vi "TestFindFaces.vi"() -> ()   [LabVIEW 2017]
uses:
  <vilib>/Enthought/Python Integration Toolkit/api/Console Visibility.ctl
  FindFaces_IMAQ.vi
  FindEyes_IMAQ.vi
  ImageFacialDetection.lvclass
  <vilib>/Enthought/Python Integration Toolkit/Python Integration Toolkit.lvlib
panel:
  in  "Tab Control":enum32{"LV Picture", "IMAQ"}(tab)
  out "image with faces":picture
  out "Image":T1(plugin-control)
  in  "Find Eyes?":bool
  out "Algorithm Time (s)":dbl
  in  "path to JPEG file":path
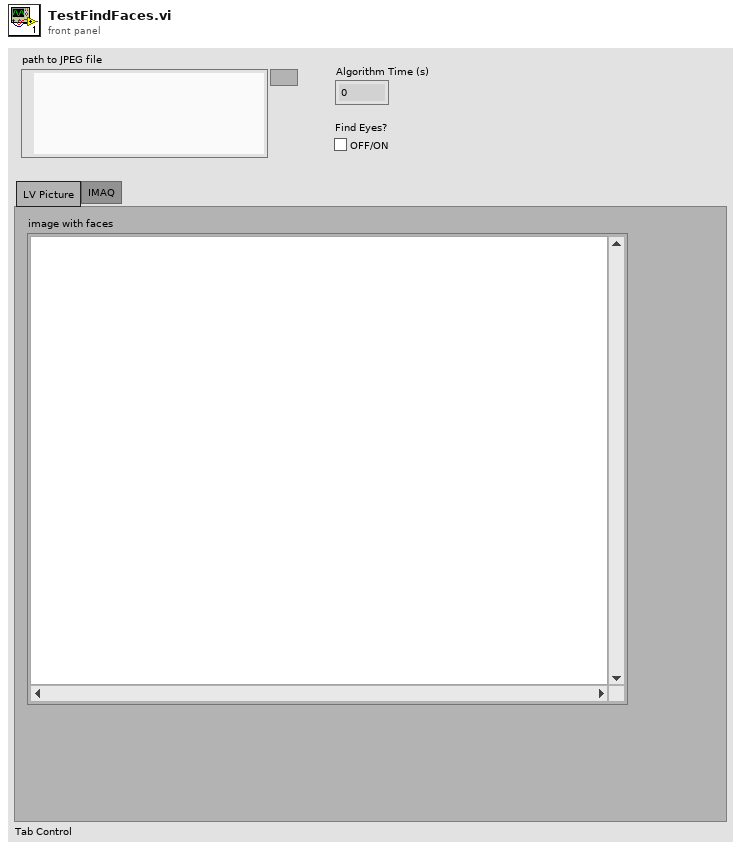
[diagram p1: front panel]
types:
  T1 = typedef "IMAQ Image.ctl" = refnum<image>
  T2 = typedef "Python Integration Toolkit.lvlib/Console Visibility.ctl" = enum16{"Show Console", "Show Console While Running", "Hide Console"}
  T3 = typedef "imagedata.ctl" = cluster{"image type":i32, "image depth":i32, "image":u8[], "mask":u8[], "colors":u32[], "Rectangle":cluster{"left":i16, "top":i16, "right":i16, "bottom":i16}}
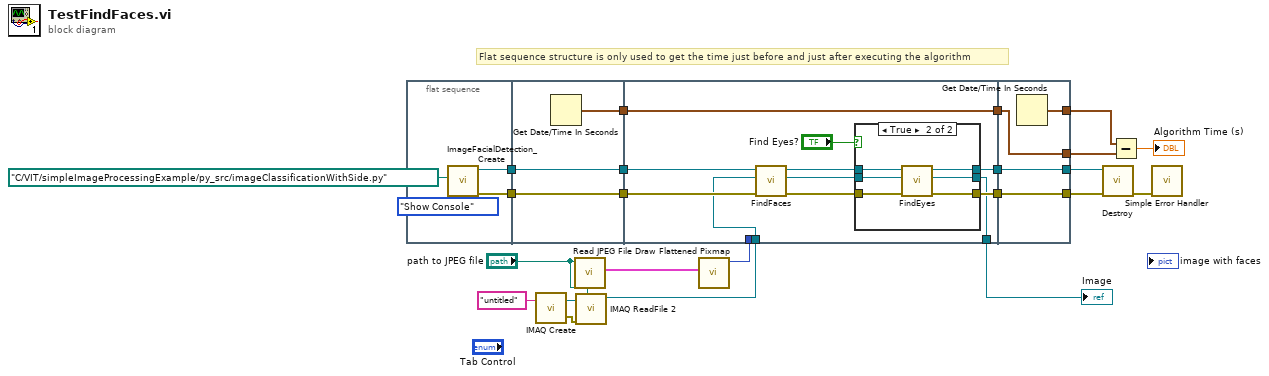
[diagram p0: block diagram]
diagram:
  # "Flat sequence structure is only used to get the time just before and just after executing the algorithm"
  n1 = flat-sequence {
    tunnel: [w25] -> w11
    tunnel: [w26] -> w9
    tunnel: w11 -> [w29]
    tunnel: [w29] -> w10
    tunnel: w9 -> [w28]
    tunnel: [w28] -> w8
    tunnel: [w27] -> w7
    tunnel: [w32] -> w2
    tunnel: w19 -> [_]
    tunnel: [w36] -> w17
    tunnel: [w34] -> w16
    tunnel: [w37] -> w15
    tunnel: w10 -> [w40]
    tunnel: w8 -> [w39]
    tunnel: w7 -> [w37]
    tunnel: w3 -> [w30]
    tunnel: [w52] -> w20
    tunnel: [w53] -> w21
    tunnel: w17 -> [w53]
    tunnel: w16 -> [w52]
    tunnel: w15 -> [w50]
    tunnel: [w51] -> w14
    tunnel: [w50] -> w13
    frame #0 {
      n2 = call "ImageFacialDetection_Create.vi"("Console visibility (hide)"=Console_Visibility."Show Console", "Path to Python Module (.py File)"=path "C:/VIT/simpleImageProcessingExample/py_src/imageClassificationWithSide.py") -> ("error out"=w26:errorcluster, "reference out"=w25:refnum<class "ImageFacialDetection.lvclass">)  [unwired: 8 in]
    }
    frame #1 {
      n3 = Get Date/Time In Seconds() -> (seconds since 1Jan1904=w27:timestamp)
    }
    frame #2 {
      n4 = call-poly "FindFaces.vi"("error in (no error)"=w39, "image"=w30, "reference in"=w40) -> ("error out"=w38:errorcluster, "image with faces"=w33:T1, "reference out"=w35:refnum<class "ImageFacialDetection.lvclass">)  [unwired: 6 in]
      n5 = case shown="True" "Find Eyes?" {
        tunnel: w38 -> [w41 w49]
        tunnel: [w41 w48] -> w36
        tunnel: w35 -> [w43 w47]
        tunnel: [w43 w46] -> w34
        tunnel: w33 -> [w42 w45]
        tunnel: [w42 w44] -> w32
        frame False {
        }
        frame True {
          n6 = call-poly "FindEyes.vi"("error in (no error)"=w49, "image"=w45, "reference in"=w47) -> ("error out"=w48:errorcluster, "image with faces"=w44:T1, "reference out"=w46:refnum<class "ImageFacialDetection.lvclass">)  [unwired: 6 in]
        }
      }
    }
    frame #3 {
      n7 = Get Date/Time In Seconds() -> (seconds since 1Jan1904=w51:timestamp)
    }
  }
  n8 = call "IMAQ Create"("Image Name"="untitled") -> ("New Image"=w6:T1, "error out"=w5:errorcluster)  [unwired: 4 in]
  n9 = call <vilib>:"Read JPEG File.vi"("path to JPEG file"="path to JPEG file") -> ("image data"=w22:T3)  [unwired: 8 in, 2 out]
  n10 = call "IMAQ ReadFile 2"("File Path"="path to JPEG file", "error in (no error)"=w5, "Image"=w6) -> ("Image Out"=w3:T1)  [unwired: 4 in, 4 out]
  n11 = call <vilib>:"Draw Flattened Pixmap.vi"("image data"=w22) -> ("new picture"=w19:picture)  [unwired: 8 in]
  n12 = call-dynamic "Destroy.vi"("error in (no error)"=w21, "reference in"=w20) -> ("error out"=w18:errorcluster)  [unwired: 8 in, 1 out]
  n13 = Subtract(x=w14, y=w13) -> (x-y=→"Algorithm Time (s)":dbl)
  n14 = call <vilib>:"Simple Error Handler.vi"("error in (no error)"=w18) -> ()  [unwired: 4 in, 5 out]
  "Image" <- w2
